vi "WriteArrDataSingleRun.vi"(6 "IndPoint":i32, 8 "error in (no error)":errorcluster caption="entrée d'erreur (pas d'erreur)", 9 "ArrDevDat":T1[](array[typedef]), 10 "Save":bool=TRUE, 11 "Interface en entrée":refnum<class "Interface.lvclass"> caption="DNL_LabVIEW Object in") -> (0 "error out":errorcluster caption="sortie d'erreur", 1 "CrvIndex":i32, 2 "CurCrvPointInd":i32, 3 "Interface en sortie":refnum<class "Interface.lvclass"> caption="DNL_LabVIEW Object out")   [LabVIEW 2019, in "Interface.lvclass"]
uses:
  Interface.lvclass
  Experiment Class/ArrDevData.ctl
  Interface.lvclass/Interface.ctl
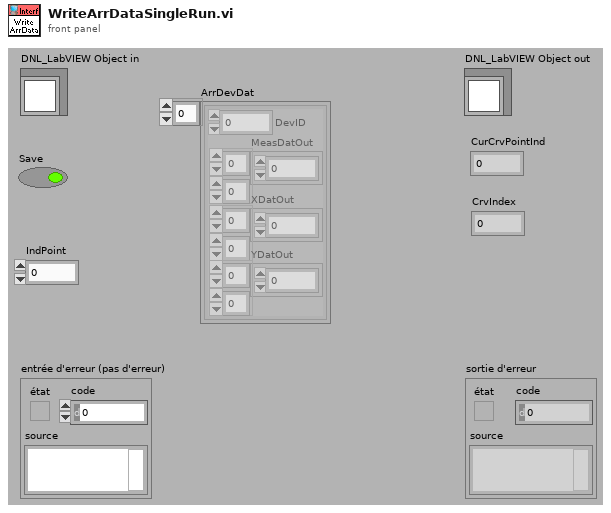
[diagram p1: front panel]
types:
  T1 = typedef "ArrDevData.ctl" = cluster{"MeasDatOut":dbl[][], "XDatOut":dbl[][], "YDatOut":dbl[][], "DevID":i32}
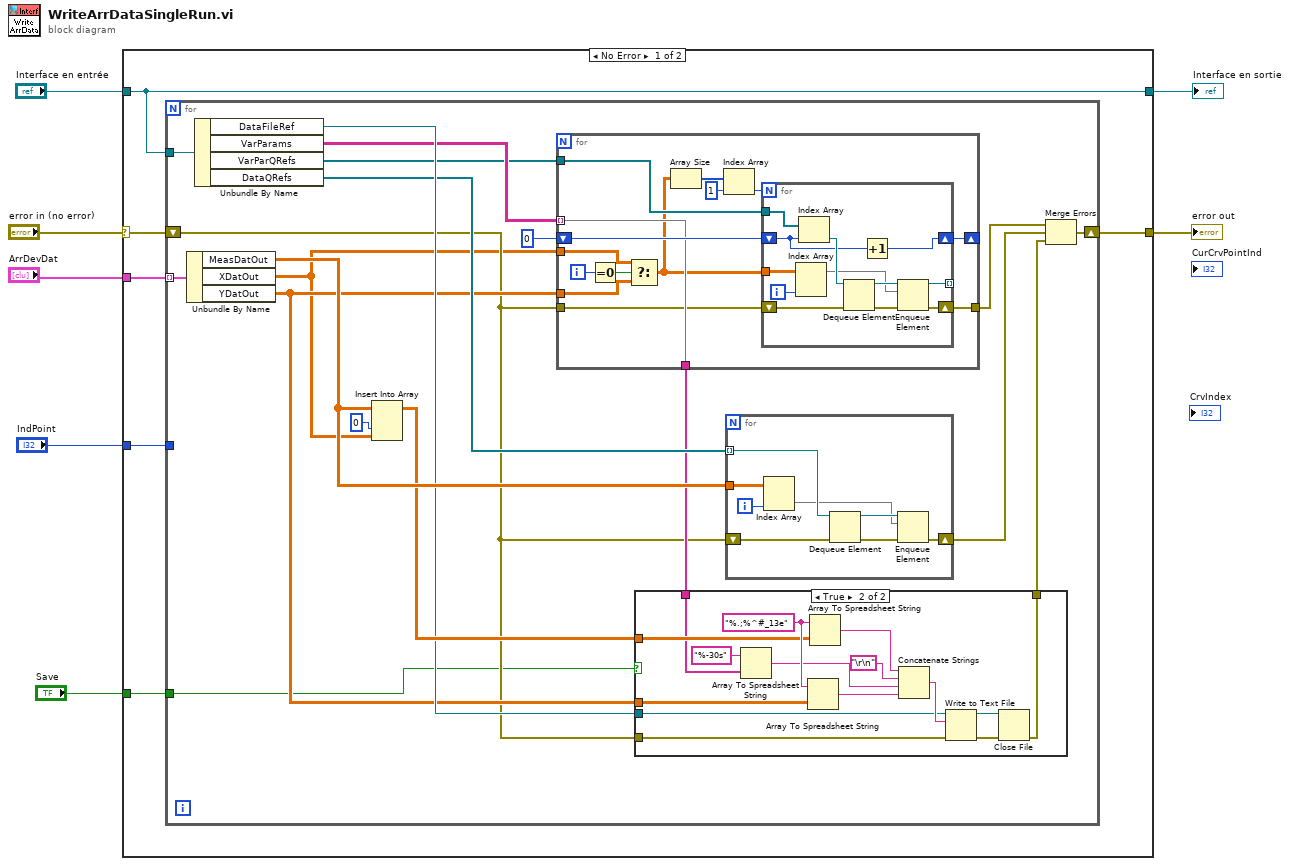
[diagram p0: block diagram]
diagram:
  n1 = case shown="No Error" "error in (no error)" {
    selector: "error in (no error)" -> [w11 w84]
    tunnel: [w10 w84] -> w6
    tunnel: [w9 w83] -> w4
    tunnel: "Interface en entrée" -> [w9 w83]
    tunnel: "IndPoint" -> [w13 _]
    tunnel: "ArrDevDat" -> [w12 _]
    tunnel: "Save" -> [w8 _]
    frame No Error {
      n2 = for {
        tunnel: w13 -> [_]
        tunnel: w9 -> [w32]
        tunnel: w12 -> [w31] mode=indexing
        shift-right: [w28] -> w10
        shift-left: w11 -> [w16]
        tunnel: w8 -> [w14]
        n3 = Unbundle By Name(w31) -> ("MeasDatOut"=w30:dbl[][], "XDatOut"=w15:dbl[][], "YDatOut"=w21:dbl[][])
        n4 = Unbundle By Name(w32) -> ("DataFileRef"=w24:refnum<file>, "VarParams"=w22:string[][], "VarParQRefs"=w20:refnum<queue>[], "DataQRefs"=w23:refnum<queue>[])
        n5 = Insert Into Array(array=w30, index (col)=0 ("indice désactivé (col)"), new element=w15) -> (w25:dbl[][])  [unwired: 1 in]
        n6 = for {
          tunnel: w22 -> [w38] mode=indexing
          tunnel: w15 -> [w42]
          tunnel: w21 -> [w41]
          tunnel: w20 -> [w46]
          tunnel: [w45] -> w19
          shift-right: [w39] -> _
          shift-left: 0 -> [w40]
          tunnel: [w38] -> w17
          tunnel: w16 -> [w37]
          i -> [w44]
          n7 = Equal To 0?(x=w44) -> (x = 0?=w43:bool)
          n8 = Select(t=w42, s=w43, f=w41) -> (s? t:f=w36:dbl[][])
          n9 = Array Size(array=w36) -> (size(s)=w35:i32[])
          n10 = Index Array(array=w35, index=1 ("indice")) -> (element=w34:i32)
          n11 = for {
            N: w34 -> [_]
            shift-right: [w56] -> w45
            shift-left: w37 -> [w55]
            tunnel: w46 -> [w54]
            tunnel: w36 -> [w52]
            shift-right: [w50] -> w39
            shift-left: w40 -> [w51]
            tunnel: [w49] -> _ mode=indexing
            i -> [w47]
            n12 = Index Array(array=w52, index (col)=w47) -> (element=w48:dbl[])  [unwired: 1 in]
            n13 = Index Array(array=w54, index=w51) -> (element=w53:refnum<queue>)
            n14 = Dequeue Element(queue=w53, error in (no error)=w55) -> (queue out=w57:refnum<queue>, error out=w58:errorcluster)  [unwired: 1 in, 2 out]
            n15 = Increment(x=w51) -> (x+1=w50:i32)
            n16 = Enqueue Element(queue=w57, element=w48, error in (no error)=w58) -> (queue out=w49:refnum<queue>, error out=w56:errorcluster)  [unwired: 1 in, 1 out]
          }
        }
        n17 = case shown="True" w14 {
          tunnel: [w67 w78] -> w26
          tunnel: w25 -> [_ w76]
          tunnel: w24 -> [_ w73]
          tunnel: w21 -> [_ w70]
          tunnel: w17 -> [_ w69]
          tunnel: w16 -> [w67 w68]
          frame False {
          }
          frame True {
            w77 = "%.;%^#_13e" ("chaîne de format")
            n18 = Array To Spreadsheet String(array=w69, 3:"%-30s" ("chaîne de format")) -> (spreadsheet string=w72:string)  [unwired: 1 in]
            n19 = Array To Spreadsheet String(array=w70, 3:w77) -> (spreadsheet string=w82:string)  [unwired: 1 in]
            n20 = Array To Spreadsheet String(array=w76, 3:w77) -> (spreadsheet string=w75:string)  [unwired: 1 in]
            n21 = Concatenate Strings(w75, "\r\n", w72, w82) -> (w81:string)
            n22 = Write to Text File(file (use dialog)=w73, text=w81, error in=w68) -> (refnum out=w79:refnum<file>, error out=w80:errorcluster)  [unwired: 1 in, 1 out]
            n23 = Close File(refnum=w79, error in=w80) -> (error out=w78:errorcluster)  [unwired: 1 out]
          }
        }
        n24 = for {
          tunnel: w30 -> [w61]
          shift-right: [w64] -> w27
          shift-left: w16 -> [w63]
          tunnel: w23 -> [w62] mode=indexing
          i -> [w59]
          n25 = Index Array(array=w61, index (col)=w59) -> (element=w60:dbl[])  [unwired: 1 in]
          n26 = Dequeue Element(queue=w62, error in (no error)=w63) -> (queue out=w65:refnum<queue>, error out=w66:errorcluster)  [unwired: 1 in, 2 out]
          n27 = Enqueue Element(queue=w65, element=w60, error in (no error)=w66) -> (error out=w64:errorcluster)  [unwired: 1 in, 2 out]
        }
        n28 = Merge Errors(w19, w27, w26) -> (w28:errorcluster)
      }
    }
    frame Error {
    }
  }
  "error out" <- w6
  "Interface en sortie" <- w4
